vi "Select App.vi"(8 "error in (no error)":errorcluster, 10 "App":refnum<class "ViaApp.lvclass">, 11 "AppListPanel in":refnum<class "AppListPanel.lvclass">) -> (0 "error out":errorcluster, 3 "AppListPanel out":refnum<class "AppListPanel.lvclass">)   [LabVIEW 2020, in "PicoG-App.lvlib" / "AppListPanel.lvclass"]
uses:
  AppListPanel.lvclass
  ViaApp/ViaApp.lvclass
  GWebAppArrayPanel/GWebAppArrayPanel.lvclass
  AppListPanel.lvclass/AppListPanel.ctl
  <vilib>/IlluminatedG/IG OOPanel/OOPanel/ArrayManager/ArrayManager.lvclass
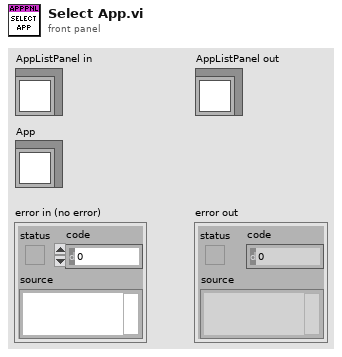
[diagram p1: front panel]
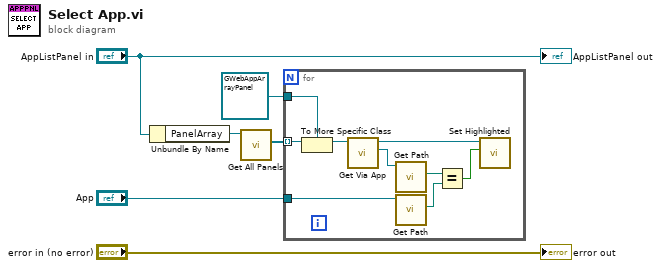
[diagram p0: block diagram]
diagram:
  n1 = Unbundle By Name("AppListPanel in") -> ("PanelArray"=w4:refnum<class "ArrayManager.lvclass">)
  n2 = call <vilib>:"Get All Panels.vi"("PanelArray in"=w4) -> ("Panels"=w3:refnum<class "ArrayPanel.lvclass">[])  [unwired: 8 in, 2 out]
  n3 = for {
    tunnel: w3 -> [w15] mode=indexing
    tunnel: "App" -> [w12]
    tunnel: refnum<class "GWebAppArrayPanel.lvclass"> refnum ("PicoG-App.lvlib:GWebAppArrayPanel.lvclass") -> [w7]
    n4 = To More Specific Class(target class=w7, reference=w15) -> (specific class reference=w14:refnum<class "GWebAppArrayPanel.lvclass">)  [unwired: 1 in, 1 out]
    n5 = call "Get Via App.vi"("GWebAppArrayPanel in"=w14) -> ("App"=w13:refnum<class "ViaApp.lvclass">, "GWebAppArrayPanel out"=w9:refnum<class "GWebAppArrayPanel.lvclass">)  [unwired: 8 in, 1 out]
    n6 = call "Get Path.vi"("ViaApp in"=w13) -> ("Path"=w11:path)  [unwired: 8 in, 2 out]
    n7 = call "Get Path.vi"("ViaApp in"=w12) -> ("Path"=w10:path)  [unwired: 8 in, 2 out]
    n8 = Equal?(x=w11, y=w10) -> (x = y?=w8:bool)
    n9 = call "Set Highlighted.vi"("Highlighted"=w8, "GWebAppArrayPanel in"=w9) -> ()  [unwired: 8 in, 2 out]
  }
  "error out" <- "error in (no error)"
  "AppListPanel out" <- "AppListPanel in"
